vi "AB_ChangeTargetFileName.vi"(8 "error in (no error)":errorcluster, 9 "Target Operating System":T1(ring), 10 "Build type":T2, 11 "Target file name":string) -> (0 "error out":errorcluster, 3 "New target file name":string)   [LabVIEW 2020]
uses:
  <vilib>/AppBuilder/AB_TargetFileType.ctl
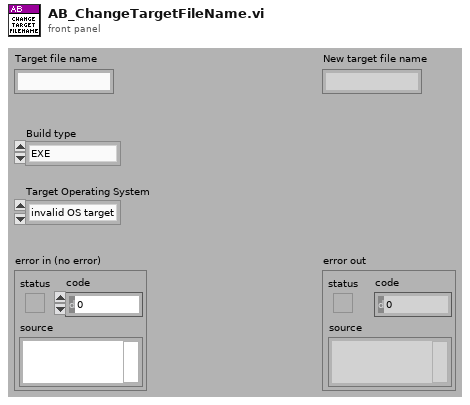
[diagram p1: front panel]
types:
  T1 = enum32{"invalid OS target", "Mac OS", "Windows 3.1", "Windows 95/NT", "Solaris 1", "Solaris 2", "HP-UX", "PowerMAX", "Linux", "Irix", "Rhapsody", "BeOS", "AIX", "OSF1", "VxWorks", "PharLap", "Carbon", "RTX", "Windows x64", "Linux x64", "Mac OS X x64"}
  T2 = typedef "AB_TargetFileType.ctl" = enum16{"EXE", "DLL", "RTEXE"}
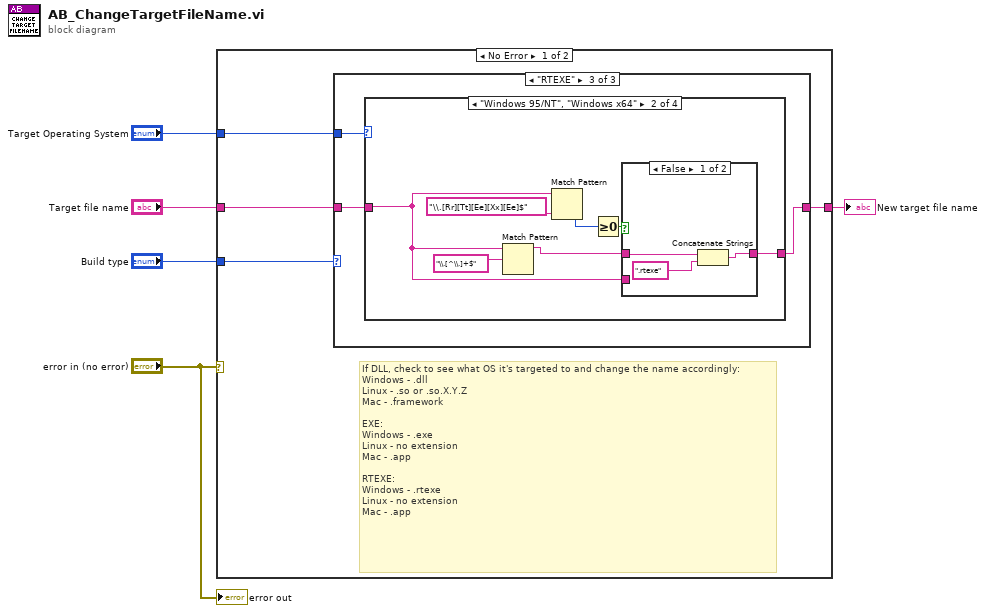
[diagram p0: block diagram]
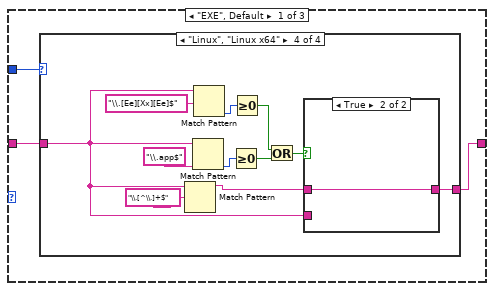
[diagram p2: hidden frame]
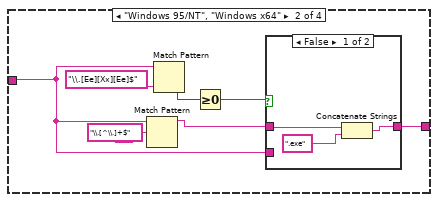
[diagram p4: hidden frame]
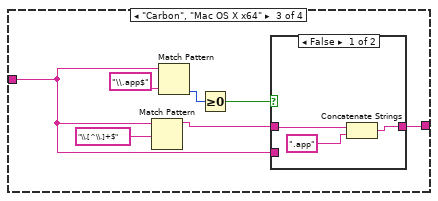
[diagram p6: hidden frame]
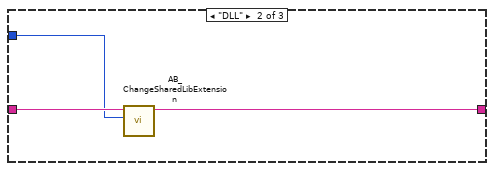
[diagram p9: hidden frame]
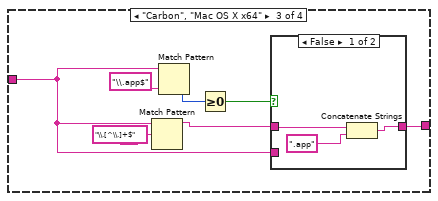
[diagram p12: hidden frame]
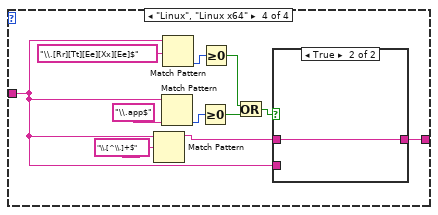
[diagram p14: hidden frame]
diagram:
  n1 = case shown="No Error" "error in (no error)" {
    tunnel: [w9 w91] -> w5
    tunnel: "Target file name" -> [w8 w91]
    tunnel: "Build type" -> [w7 _]
    tunnel: "Target Operating System" -> [w6 _]
    frame No Error {
      # "If DLL, check to see what OS it's targeted to and change the name accordingly:\nWindows - .dll\nLinux - .so or .so.X.Y.Z\nMac - .framework\n\nEXE:\nWindows - .exe\nLinux - no extension\nMac - .app\n\nRTEXE:\nWindows - .rtexe\nLinux - no extension\nMac - .app"
      n2 = case shown="\"RTEXE\"" w7 {
        tunnel: w6 -> [w12 w50 w54]
        tunnel: w8 -> [w11 w51 w53]
        tunnel: [w10 w49 w52] -> w9
        frame "EXE", Default {
          n3 = case shown="\"Linux\", \"Linux x64\"" w12 {
            tunnel: w11 -> [w13 w15 w26 w36]
            tunnel: [w13 w14 w25 w37] -> w10
            frame Default {
            }
            frame "Windows 95/NT", "Windows x64" {
              n4 = Match Pattern(string=w15, regular expression="\\.[^\\.]+$") -> (before substring=w20:string)  [unwired: 1 in, 3 out]
              n5 = Match Pattern(string=w15, regular expression="\\.[Ee][Xx][Ee]$") -> (offset past match=w17:i32)  [unwired: 1 in, 3 out]
              n6 = Greater Or Equal To 0?(x=w17) -> (x >= 0?=w16:bool)
              n7 = case shown="False" w16 {
                tunnel: w20 -> [w21 _]
                tunnel: [w22 w24] -> w14
                tunnel: w15 -> [_ w24]
                frame False {
                  n8 = Concatenate Strings(w21, ".exe" ("y")) -> (w22:string)
                }
                frame True {
                }
              }
            }
            frame "Carbon", "Mac OS X x64" {
              n9 = Match Pattern(string=w26, regular expression="\\.[^\\.]+$") -> (before substring=w31:string)  [unwired: 1 in, 3 out]
              n10 = Match Pattern(string=w26, regular expression="\\.app$") -> (offset past match=w28:i32)  [unwired: 1 in, 3 out]
              n11 = Greater Or Equal To 0?(x=w28) -> (x >= 0?=w27:bool)
              n12 = case shown="False" w27 {
                tunnel: w31 -> [w32 _]
                tunnel: [w33 w35] -> w25
                tunnel: w26 -> [_ w35]
                frame False {
                  n13 = Concatenate Strings(w32, ".app" ("y")) -> (w33:string)
                }
                frame True {
                }
              }
            }
            frame "Linux", "Linux x64" {
              n14 = Match Pattern(string=w36, regular expression="\\.[^\\.]+$") -> (before substring=w46:string)  [unwired: 1 in, 3 out]
              n15 = Match Pattern(string=w36, regular expression="\\.app$") -> (offset past match=w43:i32)  [unwired: 1 in, 3 out]
              n16 = Match Pattern(string=w36, regular expression="\\.[Ee][Xx][Ee]$") -> (offset past match=w41:i32)  [unwired: 1 in, 3 out]
              n17 = Greater Or Equal To 0?(x=w43) -> (x >= 0?=w40:bool)
              n18 = Greater Or Equal To 0?(x=w41) -> (x >= 0?=w39:bool)
              n19 = Or(x=w39, y=w40) -> (x .or. y?=w38:bool)
              n20 = case shown="True" w38 {
                tunnel: w46 -> [_ w48]
                tunnel: [w47 w48] -> w37
                tunnel: w36 -> [w47 _]
                frame False {
                }
                frame True {
                }
              }
            }
          }
        }
        frame "DLL" {
          n21 = call <vilib>:"AB_ChangeSharedLibExtension.vi"("Target OS"=w50, "Target file name"=w51) -> ("New target file name"=w49:string)  [unwired: 8 in, 1 out]
        }
        frame "RTEXE" {
          n22 = case shown="\"Windows 95/NT\", \"Windows x64\"" w54 {
            tunnel: w53 -> [w55 w57 w68 w78]
            tunnel: [w55 w56 w67 w79] -> w52
            frame Default {
            }
            frame "Windows 95/NT", "Windows x64" {
              n23 = Match Pattern(string=w57, regular expression="\\.[^\\.]+$") -> (before substring=w62:string)  [unwired: 1 in, 3 out]
              n24 = Match Pattern(string=w57, regular expression="\\.[Rr][Tt][Ee][Xx][Ee]$") -> (offset past match=w59:i32)  [unwired: 1 in, 3 out]
              n25 = Greater Or Equal To 0?(x=w59) -> (x >= 0?=w58:bool)
              n26 = case shown="False" w58 {
                tunnel: w62 -> [w63 _]
                tunnel: [w64 w66] -> w56
                tunnel: w57 -> [_ w66]
                frame False {
                  n27 = Concatenate Strings(w63, ".rtexe" ("y")) -> (w64:string)
                }
                frame True {
                }
              }
            }
            frame "Carbon", "Mac OS X x64" {
              n28 = Match Pattern(string=w68, regular expression="\\.[^\\.]+$") -> (before substring=w73:string)  [unwired: 1 in, 3 out]
              n29 = Match Pattern(string=w68, regular expression="\\.app$") -> (offset past match=w70:i32)  [unwired: 1 in, 3 out]
              n30 = Greater Or Equal To 0?(x=w70) -> (x >= 0?=w69:bool)
              n31 = case shown="False" w69 {
                tunnel: w73 -> [w74 _]
                tunnel: [w75 w77] -> w67
                tunnel: w68 -> [_ w77]
                frame False {
                  n32 = Concatenate Strings(w74, ".app" ("y")) -> (w75:string)
                }
                frame True {
                }
              }
            }
            frame "Linux", "Linux x64" {
              n33 = Match Pattern(string=w78, regular expression="\\.[^\\.]+$") -> (before substring=w88:string)  [unwired: 1 in, 3 out]
              n34 = Match Pattern(string=w78, regular expression="\\.app$") -> (offset past match=w85:i32)  [unwired: 1 in, 3 out]
              n35 = Match Pattern(string=w78, regular expression="\\.[Rr][Tt][Ee][Xx][Ee]$") -> (offset past match=w83:i32)  [unwired: 1 in, 3 out]
              n36 = Greater Or Equal To 0?(x=w85) -> (x >= 0?=w82:bool)
              n37 = Greater Or Equal To 0?(x=w83) -> (x >= 0?=w81:bool)
              n38 = Or(x=w81, y=w82) -> (x .or. y?=w80:bool)
              n39 = case shown="True" w80 {
                tunnel: w88 -> [_ w90]
                tunnel: [w89 w90] -> w79
                tunnel: w78 -> [w89 _]
                frame False {
                }
                frame True {
                }
              }
            }
          }
        }
      }
    }
    frame Error {
    }
  }
  "New target file name" <- w5
  "error out" <- "error in (no error)"
